vi "Write SafeBTE Event.vi"(8 "error in":errorcluster, 10 "SafeBTE Event":refnum<user-event>, 11 "Engine in":refnum<class "Engine.lvclass">) -> (0 "error out":errorcluster, 3 "Engine out":refnum<class "Engine.lvclass">)   [LabVIEW 2023, in "Engine.lvlib" / "Engine.lvclass"]
uses:
  Project/Engine.lvclass
  Project/Engine.lvclass/Engine.ctl
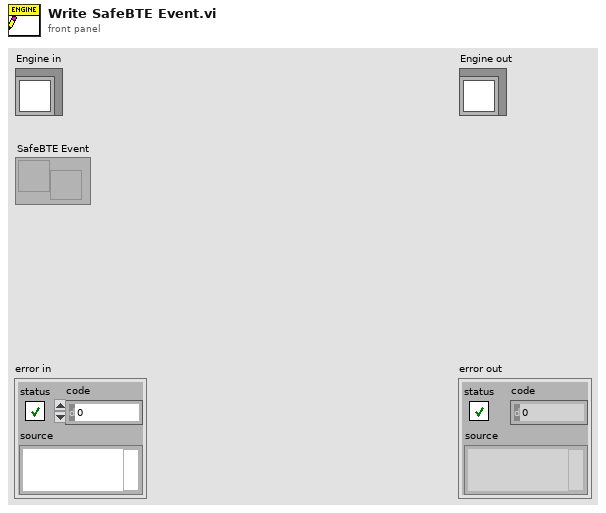
[diagram p1: front panel]
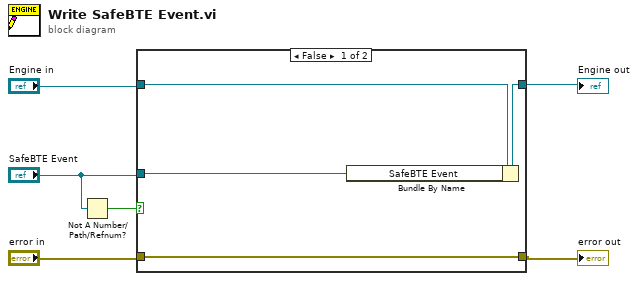
[diagram p0: block diagram]
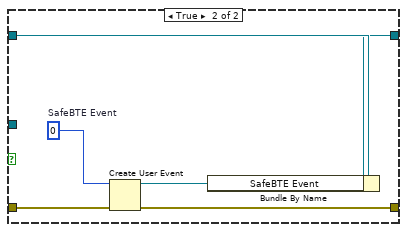
[diagram p2: hidden frame]
diagram:
  n1 = Not A Number/Path/Refnum?(number/path/refnum="SafeBTE Event") -> (NaN/Path/Refnum?=w3:bool)
  n2 = case shown="False" w3 {
    tunnel: [w7 w13] -> w2
    tunnel: [w9 w12] -> w1
    tunnel: "Engine in" -> [w10 w16]
    tunnel: "SafeBTE Event" -> [w8 _]
    tunnel: "error in" -> [w7 w14]
    frame False {
      n3 = Bundle By Name(cluster=w10, "SafeBTE Event"=w8) -> (w9:refnum<class "Engine.lvclass">)
    }
    frame True {
      w15 = 0  # SafeBTE Event
      n4 = Create User Event(user event datatype=w15, error in=w14) -> (user event=w11:refnum<user-event>, error out=w13:errorcluster)
      n5 = Bundle By Name(cluster=w16, "SafeBTE Event"=w11) -> (w12:refnum<class "Engine.lvclass">)
    }
  }
  "error out" <- w2
  "Engine out" <- w1
